vi "MC5e Unit_Manager.vi"(7 "Mode (Get)":T7, 8 "error in":errorcluster, 9 "Set In":set{T1}(c389), 10 "Unit In (Add/Replace)":T1={"Unit Fatigue Level"=enum."Not Fatigued", "Flying Unit"=FALSE, "Mounted Unit"=FALSE, "Defending from Stronghold"=FALSE, "Difficult Terrain Types"=[0, 1, 3, 6, 7], "Squads in Unit"=[], "Unit Info"={"Unit Name"="", "Unit Commander"="", "Current Morale"=0.0, "Current BR"=0.0, "Capacity %"=0.0, "Speed Mod"=0.0, "Location"={"X coordinate"=0.0, "Y coordinate"=0.0}, "Unit Notes"=""}, "Range"=0.0, "Full BR"=0.0, "Base Speed"=0.0, "Base Morale"=0.0} {"Squads in Unit"."CR" items=["30", "29", "28", "27", "26", "25", "24", "23", "22", "21", "20", "19", "18", "17", "16", "15", "14", "13", "12", "11", "10", "9", "8", "7", "6", "5", "4", "3", "2", "1", "1/2", "1/4", "1/8"]}, 11 "index (get/delete)":i32) -> (0 "error out":errorcluster, 1 "Set Out":set{T1}(c389), 2 "Unit":T1={"Unit Fatigue Level"=enum."Not Fatigued", "Flying Unit"=FALSE, "Mounted Unit"=FALSE, "Defending from Stronghold"=FALSE, "Difficult Terrain Types"=[0, 1, 3, 6, 7], "Squads in Unit"=[], "Unit Info"={"Unit Name"="", "Unit Commander"="", "Current Morale"=0.0, "Current BR"=0.0, "Capacity %"=0.0, "Speed Mod"=0.0, "Location"={"X coordinate"=0.0, "Y coordinate"=0.0}, "Unit Notes"=""}, "Range"=0.0, "Full BR"=0.0, "Base Speed"=0.0, "Base Morale"=0.0} {"Squads in Unit"."CR" items=["30", "29", "28", "27", "26", "25", "24", "23", "22", "21", "20", "19", "18", "17", "16", "15", "14", "13", "12", "11", "10", "9", "8", "7", "6", "5", "4", "3", "2", "1", "1/2", "1/4", "1/8"]}, 3 "set size":i32)   [LabVIEW 2020]
uses:
  Location.ctl
  MC5e Terrain types.ctl
  MC5e Unit.ctl
  MC5e Size_Categories.ctl
  MC5e Squad_Info.ctl
  MC5e Unit Header.ctl
  MC5e Unit_Manager_Modes.ctl
panel:
  # "Squads are restricted to one type of soldier (i.e  Archers) and all of the same level.\nIf you want mixed CR or mixed types, use multiple squads."
  # "Squads are restricted to one type of soldier (i.e  Archers) and all of the same level.\nIf you want mixed CR or mixed types, use multiple squads."
  # "Squads are restricted to one type of soldier (i.e  Archers) and all of the same level.\nIf you want mixed CR or mixed types, use multiple squads."
  # "Squads are restricted to one type of soldier (i.e  Archers) and all of the same level.\nIf you want mixed CR or mixed types, use multiple squads."
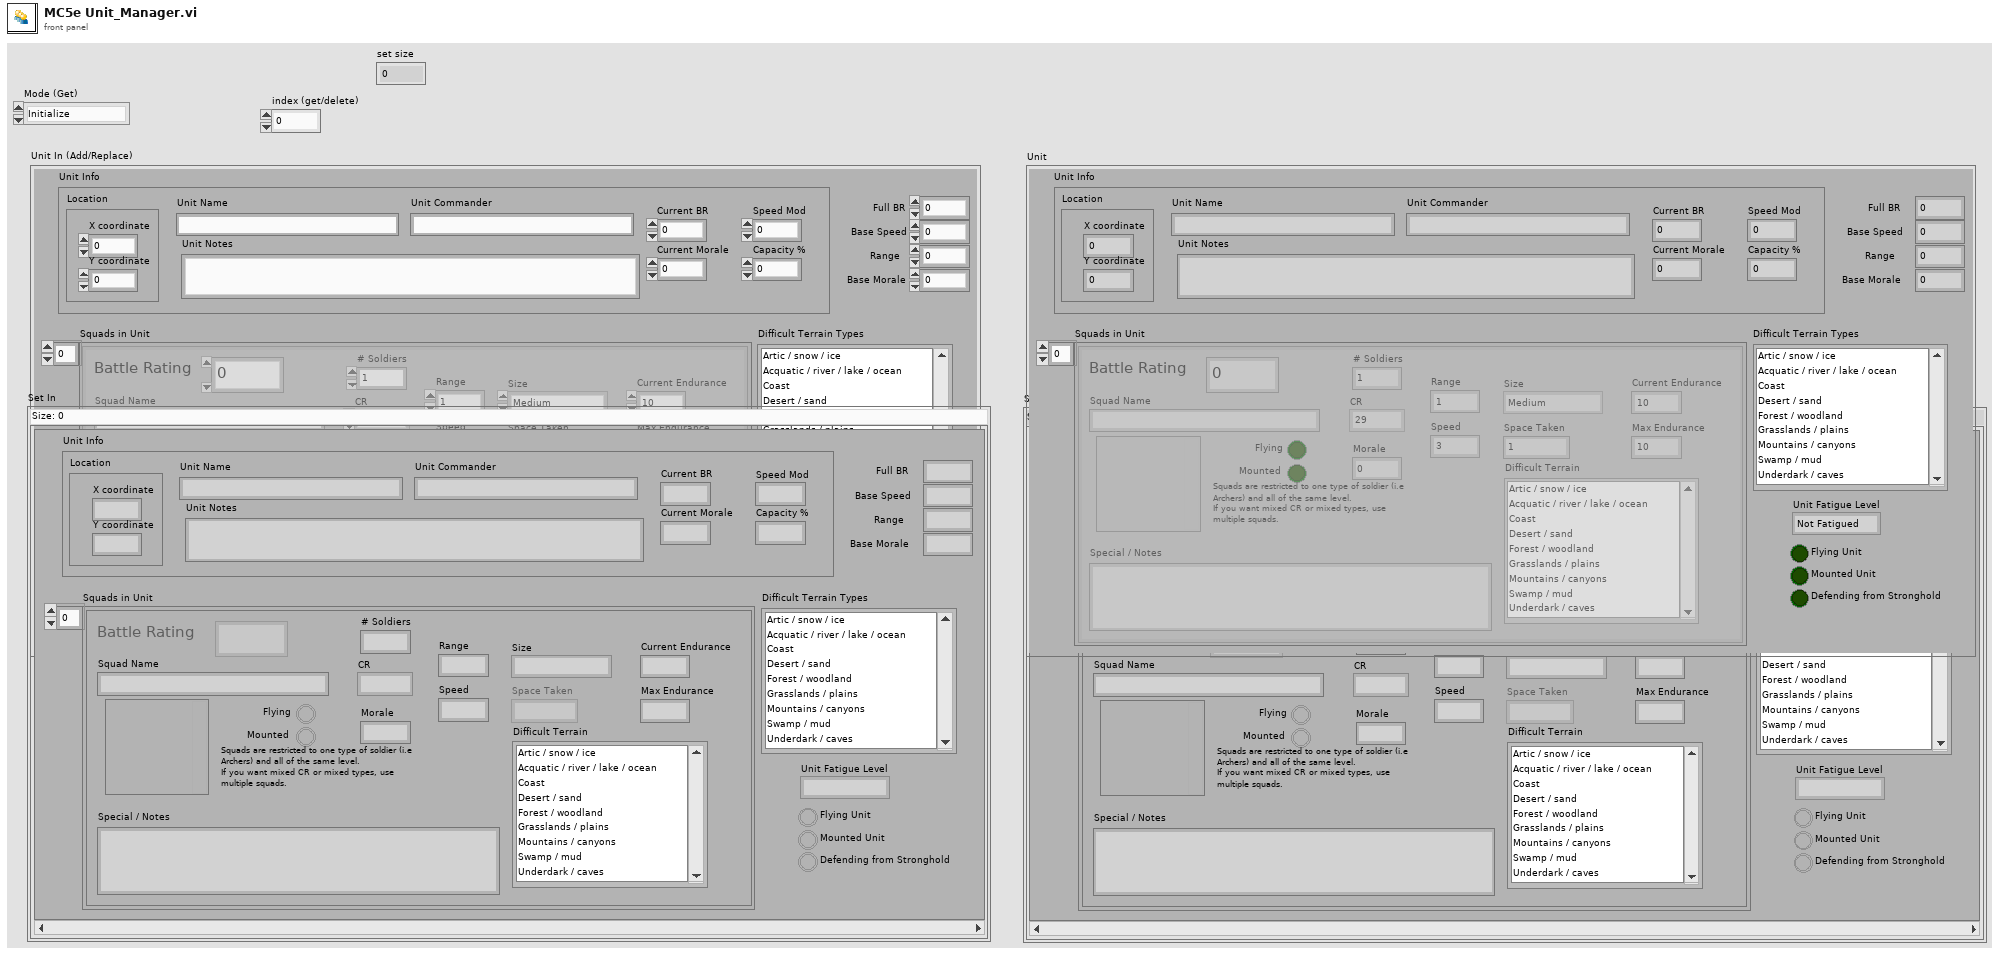
[diagram p1: front panel]
types:
  T1 = typedef "MC5e Unit.ctl" = cluster{"Unit Fatigue Level":enum16{"Not Fatigued", "Fatigued", "Seriously Fatigued"}, "Flying Unit":bool, "Mounted Unit":bool, "Defending from Stronghold":bool, "Difficult Terrain Types":T2, "Squads in Unit":T3[], "Unit Info":T5, "Range":dbl, "Full BR":dbl, "Base Speed":dbl, "Base Morale":dbl}
  T2 = typedef "MC5e Terrain types.ctl" = i32[]
  T3 = typedef "MC5e Squad_Info.ctl" = cluster{"Squad Name":string, "# Soldiers":u16, "Battle Rating":u16, "Flying":bool, "Mounted":bool, "Speed":u16, "Range":u16, "Morale":i32, "Token Image":variant, "Max Endurance":u16, "Current Endurance":i32, "Size":T4, "Space Taken":u16, "Difficult Terrain":i32[], "CR":u16, "Special / Notes":string}
  T4 = typedef "MC5e Size_Categories.ctl" = enum16{"Tiny", "Small", "Medium", "Large", "Huge", "Gargantuan"}
  T5 = typedef "MC5e Unit Header.ctl" = cluster{"Unit Name":string, "Unit Commander":string, "Current Morale":dbl, "Current BR":dbl, "Capacity %":dbl, "Speed Mod":dbl, "Location":T6, "Unit Notes":string}
  T6 = typedef "Location.ctl" = cluster{"X coordinate":dbl, "Y coordinate":dbl}
  T7 = typedef "MC5e Unit_Manager_Modes.ctl" = enum16{"Initialize", "Add Unit", "Delete Unit", "Get Unit", "Load Set"}
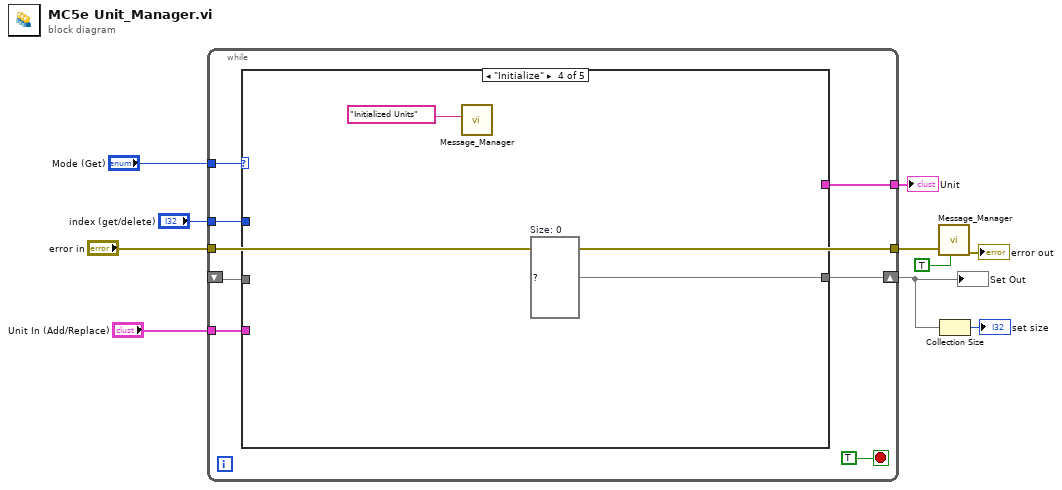
[diagram p0: block diagram]
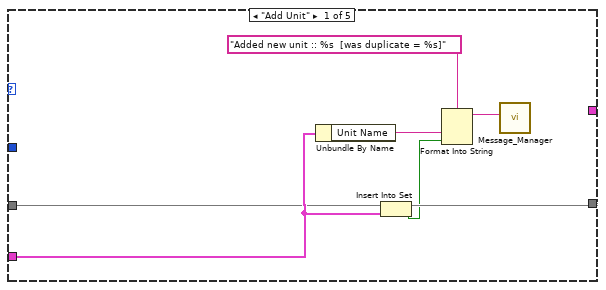
[diagram p2: hidden frame]
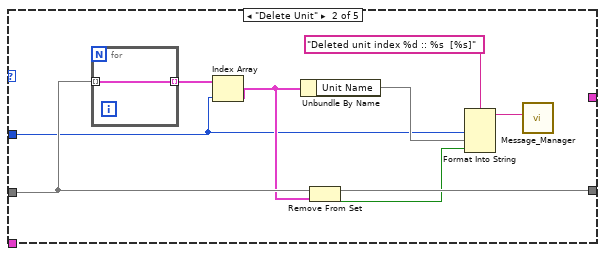
[diagram p3: hidden frame]
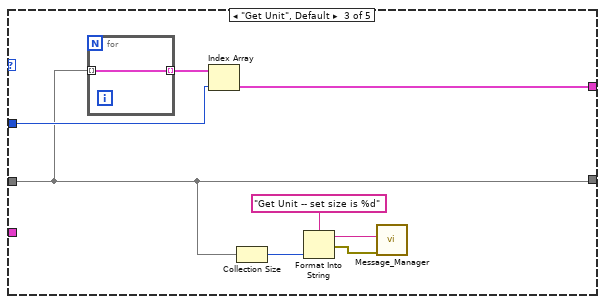
[diagram p4: hidden frame]
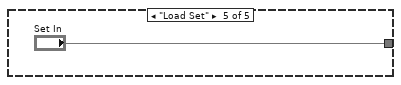
[diagram p5: hidden frame]
diagram:
  n1 = while {
    tunnel: "error in" -> [w12]
    tunnel: "Mode (Get)" -> [w17]
    shift-right: [w16] -> w5
    shift-left: _ -> [w15]
    tunnel: "index (get/delete)" -> [w14]
    tunnel: [w13] -> w1
    tunnel: [w12] -> w7
    tunnel: "Unit In (Add/Replace)" -> [w11]
    stop <- TRUE stop-if-true
    n2 = case shown="\"Initialize\"" w17 {
      tunnel: [w25 w32 w39 w45 "Set In"] -> w16
      tunnel: w15 -> [w20 w33 w39 _ _]
      tunnel: w14 -> [_ w27 w41 _ _]
      tunnel: [_ _ w42 _ _] -> w13
      tunnel: w11 -> [w21 _ _ _ _]
      frame "Add Unit" {
        n3 = Unbundle By Name(w21) -> ("Unit Name"=w19:string)
        n4 = Insert Into Set(10:w21, 11:w20) -> (2:w22:bool, 3:w25:set{T1})
        n5 = Format Into String(format string="Added new unit :: %s  [was duplicate = %s]", w19, w22) -> (resulting string=w23:string)  [unwired: 2 in, 1 out]
        n6 = call "Message_Manager.vi"("New Entry"=w23) -> ()  [unwired: 6 in, 5 out]
      }
      frame "Delete Unit" {
        n7 = for {
          tunnel: [w35] -> w34 mode=indexing
          tunnel: w33 -> [w35] mode=indexing
        }
        n8 = Index Array(array=w34, index=w27) -> (element=w28:T1)
        n9 = Unbundle By Name(w28) -> ("Unit Name"=w30)
        n10 = Remove From Set(10:w28, 11:w33) -> (2:w26:bool, 3:w32:set{T1})
        n11 = Format Into String(format string="Deleted unit index %d :: %s  [%s]", w27, w30, w26) -> (resulting string=w29:string)  [unwired: 2 in, 1 out]
        n12 = call "Message_Manager.vi"("New Entry"=w29) -> ()  [unwired: 6 in, 5 out]
      }
      frame "Get Unit", Default {
        n13 = for {
          tunnel: [w44] -> w43 mode=indexing
          tunnel: w39 -> [w44] mode=indexing
        }
        n14 = Index Array(array=w43, index=w41) -> (element=w42:T1)
        n15 = Collection Size(1:w39) -> (0:w38:i32)
        n16 = Format Into String(format string="Get Unit -- set size is %d", w38) -> (resulting string=w37:string, error out=w36:errorcluster)  [unwired: 2 in]
        n17 = call "Message_Manager.vi"("error in"=w36, "New Entry"=w37) -> ()  [unwired: 5 in, 5 out]
      }
      frame "Initialize" {
        w45 = set{T1} {}  # Size: 0
        n18 = call "Message_Manager.vi"("New Entry"="Initialized Units" ("format string")) -> ()  [unwired: 6 in, 5 out]
      }
      frame "Load Set" {
      }
    }
  }
  "Set Out" <- w5
  "Unit" <- w1
  n19 = call "Message_Manager.vi"("Log only on Err"=TRUE, "error in"=w7) -> ("error out"=→"error out":errorcluster)  [unwired: 5 in, 4 out]
  n20 = Collection Size(1:w5) -> (0:→"set size":i32)
